vi "Combined Data.vi"(8 "error in (no error)":errorcluster, 11 "Scan Data Process in":T1) -> (0 "error out":errorcluster, 3 "Scan Data Process out":T1)   [LabVIEW 2015, in "Exposure Process.lvlib"]
uses:
  Exposure Process.lvlib
  Control_Scan Data Process.ctl
  <vilib>/addons/PointValueMap/controls/PointMap.ctl
  Control_EXP Information.ctl
  Control_File Save Setup.ctl
  Control_Enable and Path.ctl
  Control_ICM Export Setting.ctl
  <vilib>/addons/PointValueMap/PointValueMap.lvlib
panel:
  out "Combined CSV Data":string[][](array[string])
  out "Combined Waveforms":waveform(dbl)[](array[waveform])
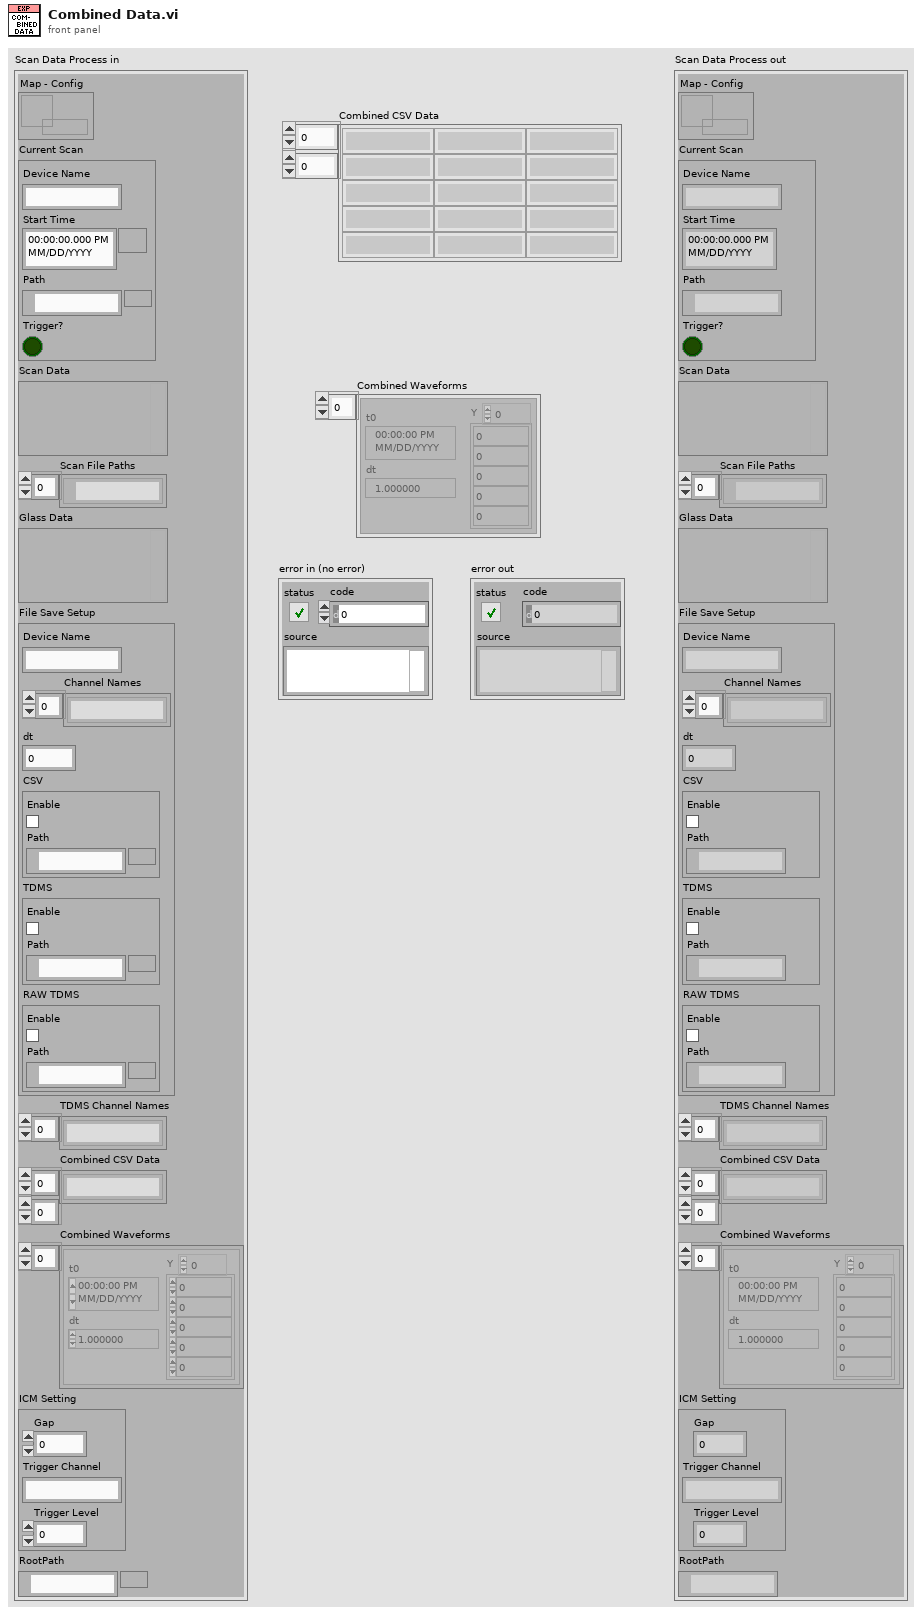
[diagram p1: front panel]
types:
  T1 = typedef "Exposure Process.lvlib/Control_Scan Data Process.ctl" = cluster{"Map - Config":T2, "Current Scan":T3, "Scan Data":variant, "Scan File Paths":path[], "Glass Data":variant, "File Save Setup":T4, "TDMS Channel Names":string[], "Combined CSV Data":string[][], "Combined Waveforms":waveform(dbl)[], "ICM Setting":T6, "RootPath":path}
  T2 = typedef "PointValueMap.lvlib/PointMap.ctl" = refnum<data-value>
  T3 = typedef "Exposure Process.lvlib/Control_EXP Information.ctl" = cluster{"Device Name":string, "Start Time":timestamp, "Path":path, "Trigger?":bool}
  T4 = typedef "Exposure Process.lvlib/Control_File Save Setup.ctl" = cluster{"Device Name":string, "Channel Names":string[], "dt":dbl, "CSV":T5, "TDMS":T5, "RAW TDMS":T5}
  T5 = typedef "Exposure Process.lvlib/Control_Enable and Path.ctl" = cluster{"Enable":bool, "Path":path}
  T6 = typedef "Exposure Process.lvlib/Control_ICM Export Setting.ctl" = cluster{"Gap":dbl, "Trigger Channel":string, "Trigger Level":dbl}
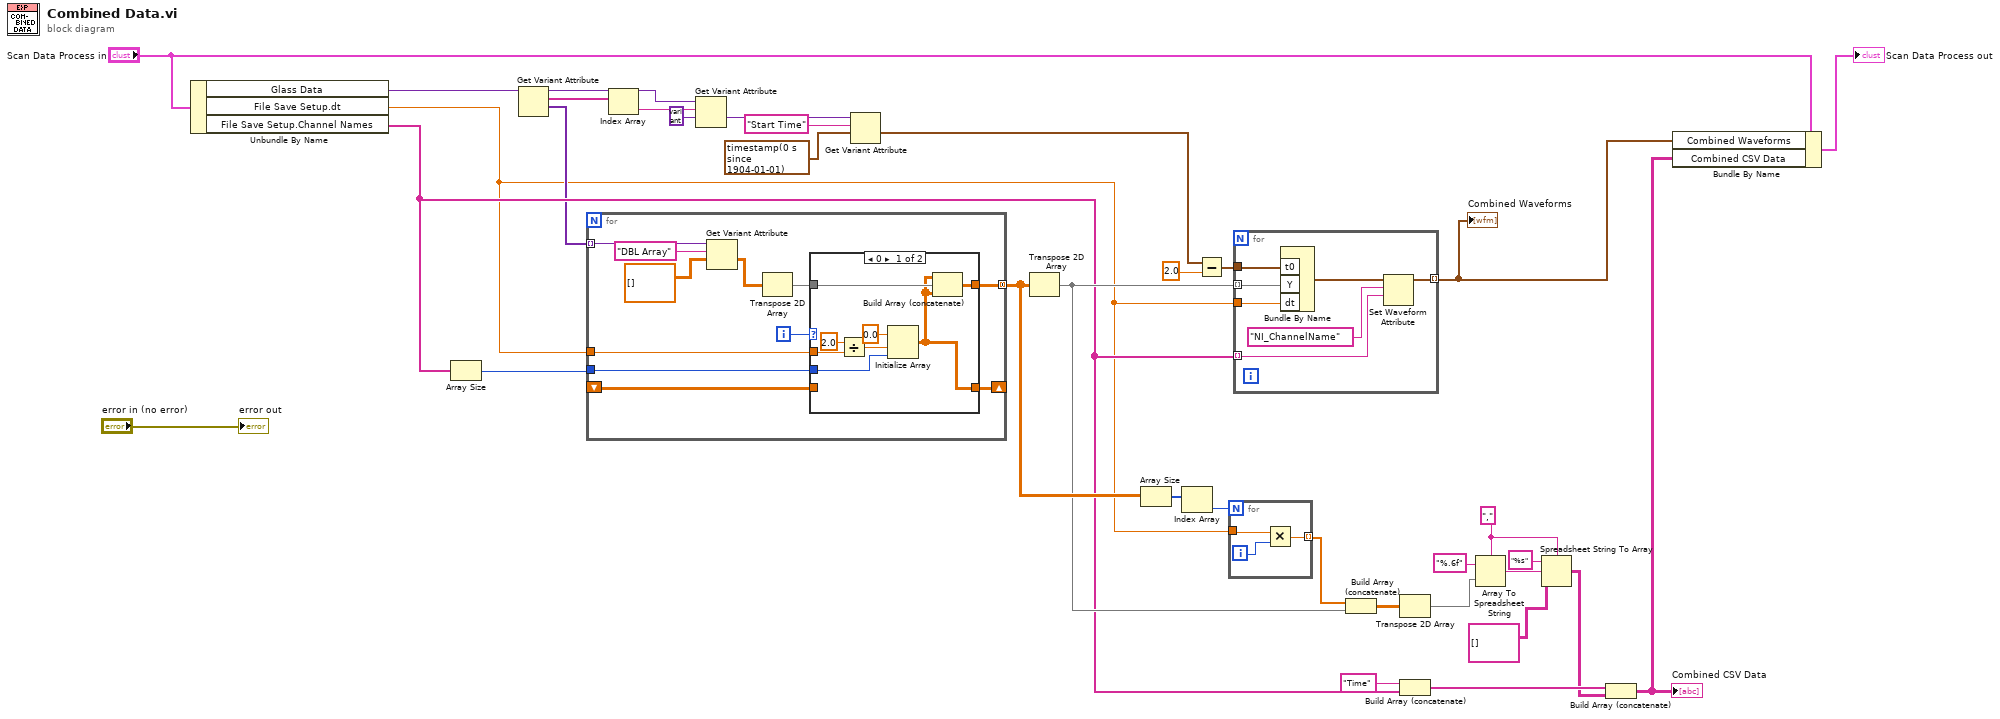
[diagram p0: block diagram]
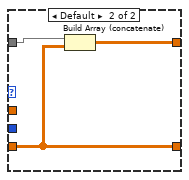
[diagram p2: hidden frame]
diagram:
  w24 = "," ("delimiter (Tab)")
  n1 = Unbundle By Name("Scan Data Process in") -> ("Glass Data"=w16:variant, "File Save Setup.dt"=w8:dbl, "File Save Setup.Channel Names"=w17:string[])
  n2 = Array Size(array=w17) -> (size(s)=w18:i32)
  n3 = Get Variant Attribute(Variant=w16) -> (duplicate Variant=w12:variant, names=w14:string[], values=w15:variant[])  [unwired: 3 in, 1 out]
  n4 = for {
    tunnel: w15 -> [w39] mode=indexing
    shift-right: [w44] -> _
    shift-left: _ -> [w43]
    tunnel: w8 -> [w42]
    tunnel: w18 -> [w41]
    tunnel: [w40] -> w21 mode=concatenating
    i -> [w45]
    n5 = Get Variant Attribute(Variant=w39, name="DBL Array", default value (empty Variant)=dbl[][] []) -> (value=w36:dbl[][])  [unwired: 1 in, 3 out]
    n6 = Transpose 2D Array(2D array=w36) -> (transposed array=w46:dbl[][])
    n7 = case shown="0" w45 {
      tunnel: w46 -> [w48 w56]
      tunnel: [w49 w57] -> w40
      tunnel: w42 -> [w54 _]
      tunnel: w41 -> [w51 _]
      tunnel: [w47 w55] -> w44
      tunnel: w43 -> [_ w55]
      frame 0 {
        n8 = Divide(x=2.0, y=w54) -> (x/y=w52:dbl)
        n9 = Initialize Array(0.0 ("element"), w52, w51) -> (w47:dbl[][])
        n10 = Build Array (concatenate)(w47, w48, w47) -> (w49:dbl[][])
      }
      frame Default {
        n11 = Build Array (concatenate)(w56, w55) -> (w57:dbl[][])
      }
    }
  }
  n12 = Index Array(array=w14) -> (element=w13:string)  [unwired: 1 in]
  n13 = Get Variant Attribute(Variant=w12, name=w13, default value (empty Variant)=variant) -> (value=w10:variant)  [unwired: 1 in, 3 out]
  n14 = Get Variant Attribute(Variant=w10, name="Start Time", default value (empty Variant)=timestamp(0 s since 1904-01-01)) -> (value=w6:timestamp)  [unwired: 1 in, 3 out]
  n15 = Transpose 2D Array(2D array=w21) -> (transposed array=w19:dbl[][])
  n16 = Array Size(array=w21) -> (size(s)=w33:i32[])
  n17 = Index Array(array=w33) -> (element=w20:i32)  [unwired: 1 in]
  n18 = Subtract(x=w6, y=2.0 ("x")) -> (x-y=w35:timestamp)
  n19 = for {
    N: w20 -> [_]
    tunnel: w8 -> [w60]
    tunnel: [w58] -> w32 mode=indexing
    i -> [w59]
    n20 = Multiply(x=w60, y=w59) -> (x*y=w58:dbl)
  }
  n21 = for {
    tunnel: w35 -> [w67]
    tunnel: w19 -> [w66] mode=indexing
    tunnel: w8 -> [w65]
    tunnel: w17 -> [w62] mode=indexing
    tunnel: [w61] -> w4 mode=indexing
    n22 = Bundle By Name("t0"=w67, "Y"=w66, "dt"=w65) -> (w64:waveform(dbl))  [unwired: 1 in]
    n23 = Set Waveform Attribute(5:w62, 6:"NI_ChannelName" ("name"), 7:w64) -> (3:w61:waveform(dbl))  [unwired: 1 in, 2 out]
  }
  "Combined Waveforms" <- w4
  n24 = Build Array (concatenate)(w32, w19) -> (w31:dbl[][])
  n25 = Transpose 2D Array(2D array=w31) -> (transposed array=w29:dbl[][])
  n26 = Build Array (concatenate)("Time", w17) -> (w23:string[])
  n27 = Array To Spreadsheet String(delimiter (Tab)=w24, array=w29, 3:"%.6f" ("format string")) -> (spreadsheet string=w27:string)
  n28 = Spreadsheet String To Array(delimiter (Tab)=w24, format string="%s", spreadsheet string=w27, array type (2D Dbl)=string[][] []) -> (array=w22:string[][])
  n29 = Build Array (concatenate)(w23, w22) -> (w3:string[][])
  "Combined CSV Data" <- w3
  n30 = Bundle By Name(cluster="Scan Data Process in", "Combined Waveforms"=w4, "Combined CSV Data"=w3) -> (→"Scan Data Process out":T1)
  "error out" <- "error in (no error)"
